vi "grid_adjust_z_piezo_pos.vi"(8 "Error in (no error)":errorcluster, 11 "Application ref in":refnum<vi>) -> (0 "Error out":errorcluster, 3 "Application ref out":refnum<vi>)   [LabVIEW 2014]
uses:
  <userlib>/Nanonis Prog Interface V5/Nanonis Prog Interface.lvlib
panel:
  in  "Amplitude (V) (NaN=no change)":sgl=180.0
  out "Z position (m)":sgl=-1.04743926e-07 format="%#_6p"
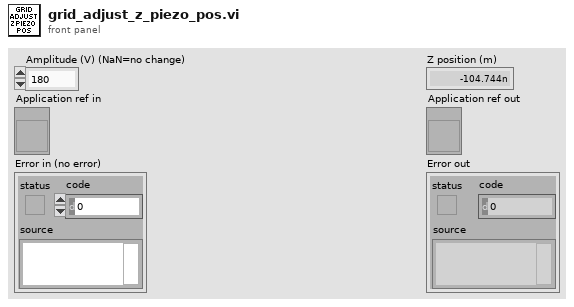
[diagram p1: front panel]
types:
  T1 = enum8{"Group 1", "Group 2", "Group 3", "Group 4", "Group 5", "Group 6"}
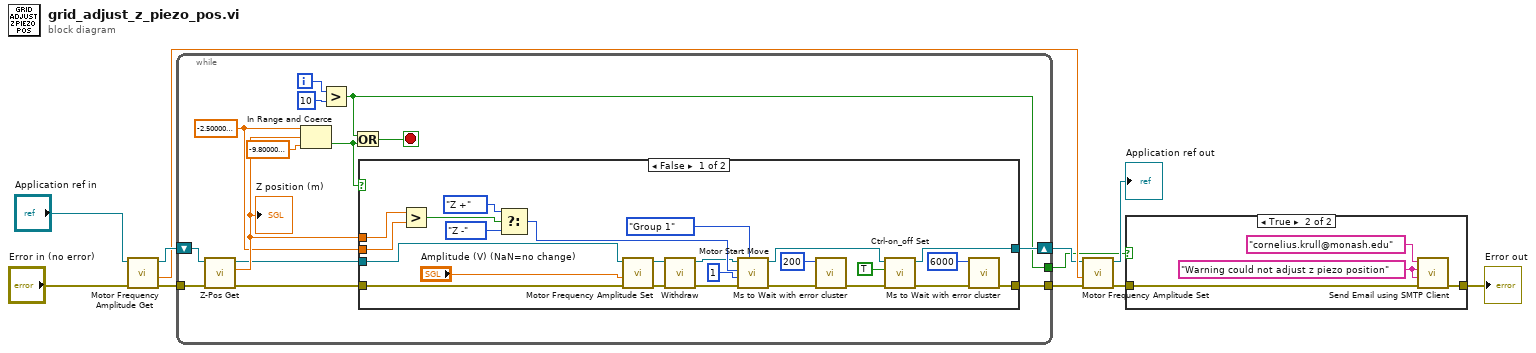
[diagram p0: block diagram]
diagram:
  n1 = call <userlib>:"Motor Frequency Amplitude Get.vi"("Error in (no error)"="Error in (no error)", "Application ref in"="Application ref in") -> ("Error out"=w10:errorcluster, "Amplitude (V)"=w9:sgl, "Application ref out"=w11:refnum<vi>)  [unwired: 6 in, 1 out]
  n2 = while {
    tunnel: w10 -> [w22]
    shift-right: [w21] -> w8
    shift-left: w11 -> [w23]
    tunnel: [w17] -> w7
    tunnel: [w12] -> w1
    i -> [w14]
    stop <- w15 stop-if-true
    w19 = sgl -2.5e-08 ("upper limit")
    n3 = call <userlib>:"Z-Pos Get.vi"("error in (no error)"=w22, "Application ref in"=w23) -> ("error out"=w16:errorcluster, "Z position (m)"=w25:sgl, "Application ref out"=w24:refnum<vi>)  [unwired: 7 in]
    "Z position (m)" <- w25
    n4 = In Range and Coerce(upper limit=w19, x=w25, lower limit=sgl -9.8e-08) -> (In Range?=w18:bool)  [unwired: 1 out]
    n5 = Greater?(x=w14, y=10) -> (0:w12:bool)
    n6 = Or(x=w12, y=w18) -> (x .or. y?=w15:bool)
    n7 = case shown="False" w18 {
      tunnel: w25 -> [w49 _]
      tunnel: w19 -> [w48 _]
      tunnel: w24 -> [w47 w51]
      tunnel: [w29 w51] -> w21
      tunnel: [w30 w50] -> w17
      tunnel: w16 -> [w28 w50]
      frame False {
        n8 = Greater?(x=w49, y=w48) -> (0:w44:bool)
        n9 = Select(t=enum16{"X +", "X -", "Y +", "Y -", "Z +", "Z -"}."Z +" ("Direction"), s=w44, f=enum16{"X +", "X -", "Y +", "Y -", "Z +", "Z -"}."Z -" ("Direction")) -> (s? t:f=w40:enum16{"X +", "X -", "Y +", "Y -", "Z +", "Z -"})
        n10 = call <userlib>:"Motor Frequency Amplitude Set.vi"("Error in (no error)"=w28, "Amplitude (V) (NaN=no change)"="Amplitude (V) (NaN=no change)", "Application ref in"=w47) -> ("Error out"=w27:errorcluster, "Application ref out"=w35:refnum<vi>)  [unwired: 7 in]
        n11 = call <userlib>:"Withdraw.vi"("Error in (no error)"=w27, "Application ref in"=w35) -> ("Error out"=w39:errorcluster, "Application ref out"=w38:refnum<vi>)  [unwired: 8 in]
        n12 = call <userlib>:"Motor Start Move.vi"("Group"=T1."Group 1", "Error in (no error)"=w39, "Number of steps"=u16 1, "Direction"=w40, "Application ref in"=w38) -> ("Error out"=w34:errorcluster, "Application ref out"=w37:refnum<vi>)  [unwired: 4 in]
        n13 = call <userlib>:"Ms to Wait with error cluster.vi"("error in (no error)"=w34, "milliseconds to wait"=u32 200) -> ("error out"=w33:errorcluster)  [unwired: 4 in, 1 out]
        n14 = call <userlib>:"Ctrl-on_off Set.vi"("error in (no error)"=w33, "Z Controller ON/OFF"=TRUE, "Application ref in"=w37) -> ("error out"=w31:errorcluster, "Application ref out"=w29:refnum<vi>)  [unwired: 7 in]
        n15 = call <userlib>:"Ms to Wait with error cluster.vi"("error in (no error)"=w31, "milliseconds to wait"=u32 6000) -> ("error out"=w30:errorcluster)  [unwired: 4 in, 1 out]
      }
      frame True {
      }
    }
  }
  n16 = call <userlib>:"Motor Frequency Amplitude Set.vi"("Error in (no error)"=w7, "Amplitude (V) (NaN=no change)"=w9, "Application ref in"=w8) -> ("Error out"=w3:errorcluster, "Application ref out"=→"Application ref out":refnum<vi>)  [unwired: 7 in]
  n17 = case shown="True" w1 {
    tunnel: w3 -> [w52 w54]
    tunnel: [w52 w53] -> w2
    frame False {
    }
    frame True {
      w55 = "Warning could not adjust z piezo position" ("Subject")
      n18 = call "Send Email using SMTP Client.vi"("error in (no error)"=w54, "Message"=w55, "Subject"=w55, "To:"="cornelius.krull@monash.edu") -> ("error out"=w53:errorcluster)  [unwired: 7 in]
    }
  }
  "Error out" <- w2
